vi "data.vi"() -> ()   [LabVIEW 2016]
uses:
  <vilib>/Analysis/NI_AALPro.lvlib
panel:
  out "output cluster":cluster{dbl[], dbl[], dbl[]}
  in  "parameter bounds":T1={"amp min"=-inf, "amp max"=inf, "damping min"=-inf, "damping max"=inf, "offset min"=0.0, "offset max"=0.0}
  out "XY Graph":cluster{dbl[], "Best Exponential Fit":dbl[]}(graph)
  out "Chopped":cluster{dbl[], dbl[]}[](graph)
  out "Lockin 4":cluster{"Y":dbl[], "Y":dbl[]}(graph)
  in  "X":cluster{"Y":dbl[], "Y":dbl[]}[](graph)=[{"Y"=array[16599 elements], "Y"=array[16599 elements]}, {"Y"=array[16599 elements], "Y"=array[16599 elements]}, {"Y"=array[16599 elements], "Y"=array[16599 elements]}, {"Y"=array[16599 elements], "Y"=array[16599 elements]}, {"Y"=array[16599 elements], "Y"=array[16599 elements]}, {"Y"=array[16599 elements], "Y"=array[16599 elements]}, {"Y"=array[16599 elements], "Y"=array[16599 elements]}, {"Y"=array[16599 elements], "Y"=array[16599 elements]}]
  # "a"
  # "d"
  # "a*exp(d*t)+c"
  # "c"
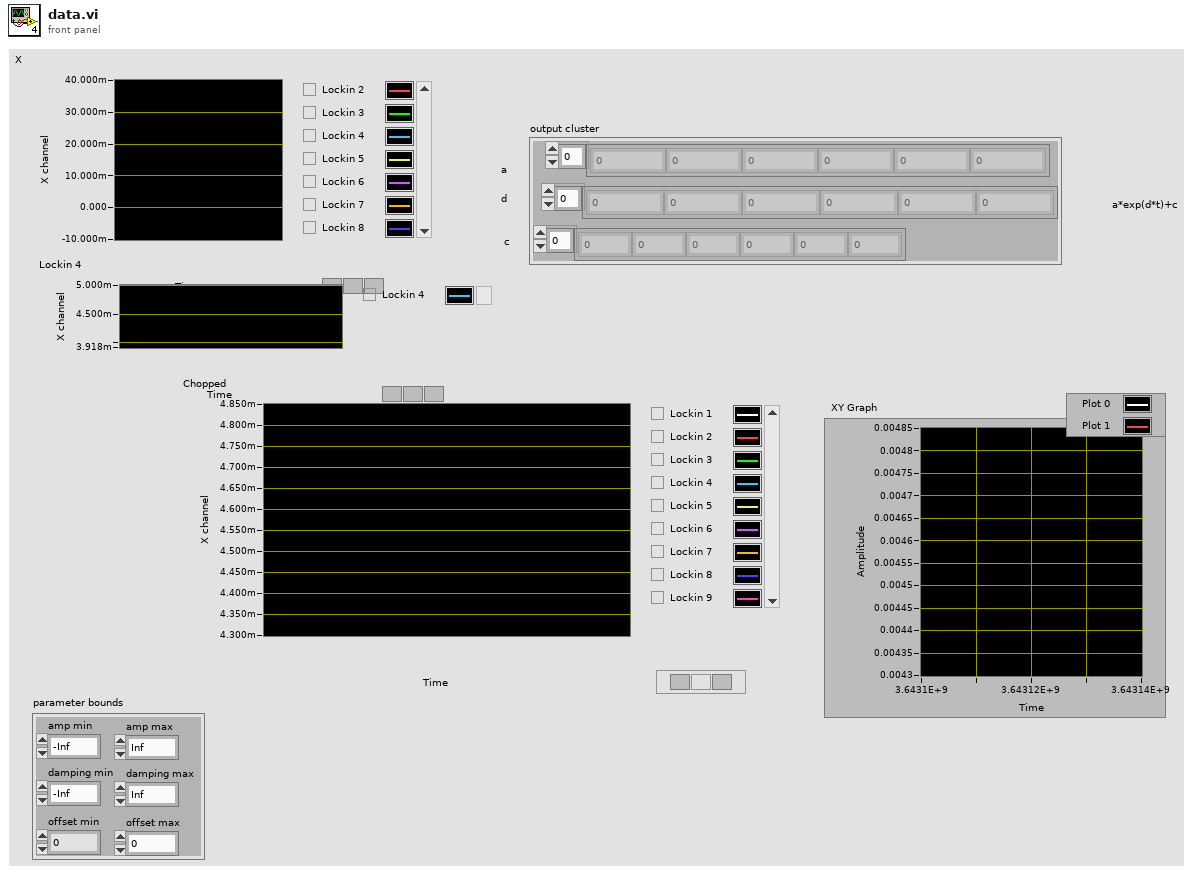
[diagram p1: front panel]
types:
  T1 = cluster{"amp min":dbl, "amp max":dbl, "damping min":dbl, "damping max":dbl, "offset min":dbl, "offset max":dbl}
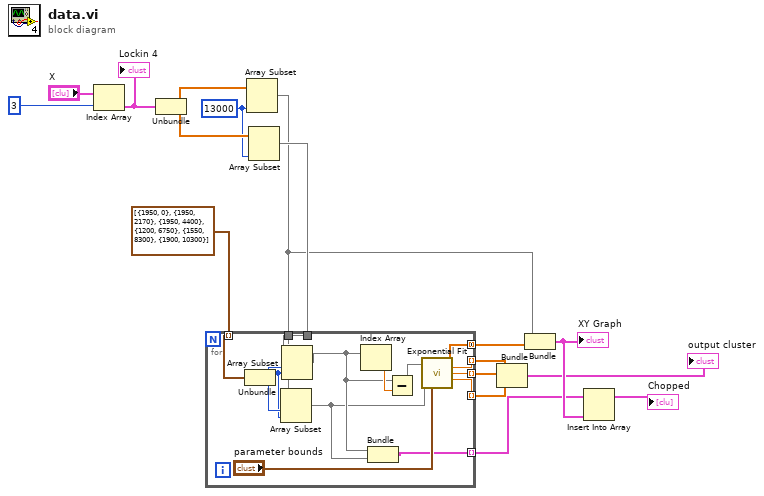
[diagram p0: block diagram]
diagram:
  w12 = 13000 ("length")
  n1 = Index Array(array="X", index=3) -> (element=w15:cluster{"Y":dbl[], "Y":dbl[]})
  "Lockin 4" <- w15
  n2 = Unbundle(w15) -> ("Y"=w14:dbl[], "Y"=w13:dbl[])
  n3 = Array Subset(array=w14, length=w12) -> (w9:dbl[])  [unwired: 1 in]
  n4 = Array Subset(array=w13, length=w12) -> (w10:dbl[])  [unwired: 1 in]
  n5 = for {
    tunnel: cluster{i32, i32}[] [{1950, 0}, {1950, 2170}, {1950, 4400}, {1200, 6750}, {1550, 8300}, {1900, 10300}] -> [w29] mode=indexing
    tunnel: w10 -> [w25]
    tunnel: w9 -> [w26]
    tunnel: [w24] -> w4 mode=indexing
    tunnel: [w23] -> w3 mode=indexing
    tunnel: [w22] -> w2 mode=indexing
    tunnel: [w21] -> w8 mode=concatenating
    tunnel: [w18] -> w6 mode=indexing
    n6 = Unbundle(w29) -> (w27:i32, w28:i32)
    n7 = Array Subset(array=w25, index=w28, length=w27) -> (w19:dbl[])
    n8 = Array Subset(array=w26, index=w28, length=w27) -> (w20:dbl[])
    n9 = Index Array(array=w20) -> (element=w31:dbl)  [unwired: 1 in]
    n10 = Bundle(w20, w19) -> (w18:cluster{dbl[], dbl[]})  [unwired: 1 in]
    n11 = Subtract(x=w20, y=w31) -> (x-y=w30:dbl[])
    n12 = call <vilib>:"Exponential Fit.vi"("Y"=w19, "X"=w30, "parameter bounds"="parameter bounds") -> ("Best Exponential Fit"=w21:dbl[], "amplitude"=w24:dbl, "damping"=w23:dbl, "offset"=w22:dbl)  [unwired: 7 in, 2 out]
  }
  n13 = Bundle(w4, w3, w2) -> (→"output cluster":cluster{dbl[], dbl[], dbl[]})  [unwired: 1 in]
  n14 = Bundle(w9, "Best Exponential Fit"=w8) -> (w7:cluster{dbl[], "Best Exponential Fit":dbl[]})  [unwired: 1 in]
  "XY Graph" <- w7
  n15 = Insert Into Array(array=w6, new element=w7) -> (→"Chopped":cluster{dbl[], dbl[]}[])  [unwired: 1 in]
